vi "Axsun GUI.vi"() -> ()   [LabVIEW 2018]
uses:
  cluster_Axsun.ctl
  General/Controls/Queue Manager Actions.ctl
  General/Controls/MessagePacket.ctl
  Axsun action.ctl
panel:
  in  "stop":bool
  out "error out":errorcluster
  out "output cluster":T1={"device array"=[], "control version"="", "Serial num"="A18009851", "LaserONTime"=0, "wave length\nat trigger"=0.0, "System status"=0.0, "clock delay"=0}
  in  "Source OFF":bool
  in  "Source ON":bool
  in  "Laser OFF":bool
  in  "Laser ON":bool
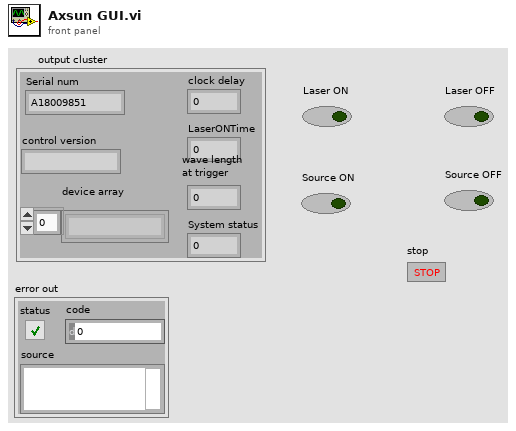
[diagram p1: front panel]
types:
  T1 = typedef "cluster_Axsun.ctl" = cluster{"device array":string[], "control version":string, "Serial num":string, "LaserONTime":i32, "wave length\nat trigger":dbl, "System status":dbl, "clock delay":u32}
  T2 = typedef "MessagePacket.ctl" = cluster{"Message":string, "Parameter":variant}
  T3 = typedef "Queue Manager Actions.ctl" = enum16{"Init", "Enqueue", "Enqueue All", "Preview Queue", "Dequeue", "Get Status", "Flush Queue", "Flush All Queues", "Release All Queues", "Release Queue", "Enqueue at Opposite End"}
  T4 = typedef "Axsun action.ctl" = enum16{"GetSystemStatus", "Clock delay", "GetLaserOnTime", "GetWaveLengthAtSweptTrigger", "Source current ON", "GetSerialNum", "GetControlVersion", "Laser ON", "Laser OFF", "Source current OFF", "Get laser handle", "Start Network Control Interface", "stop", "Create handle"}
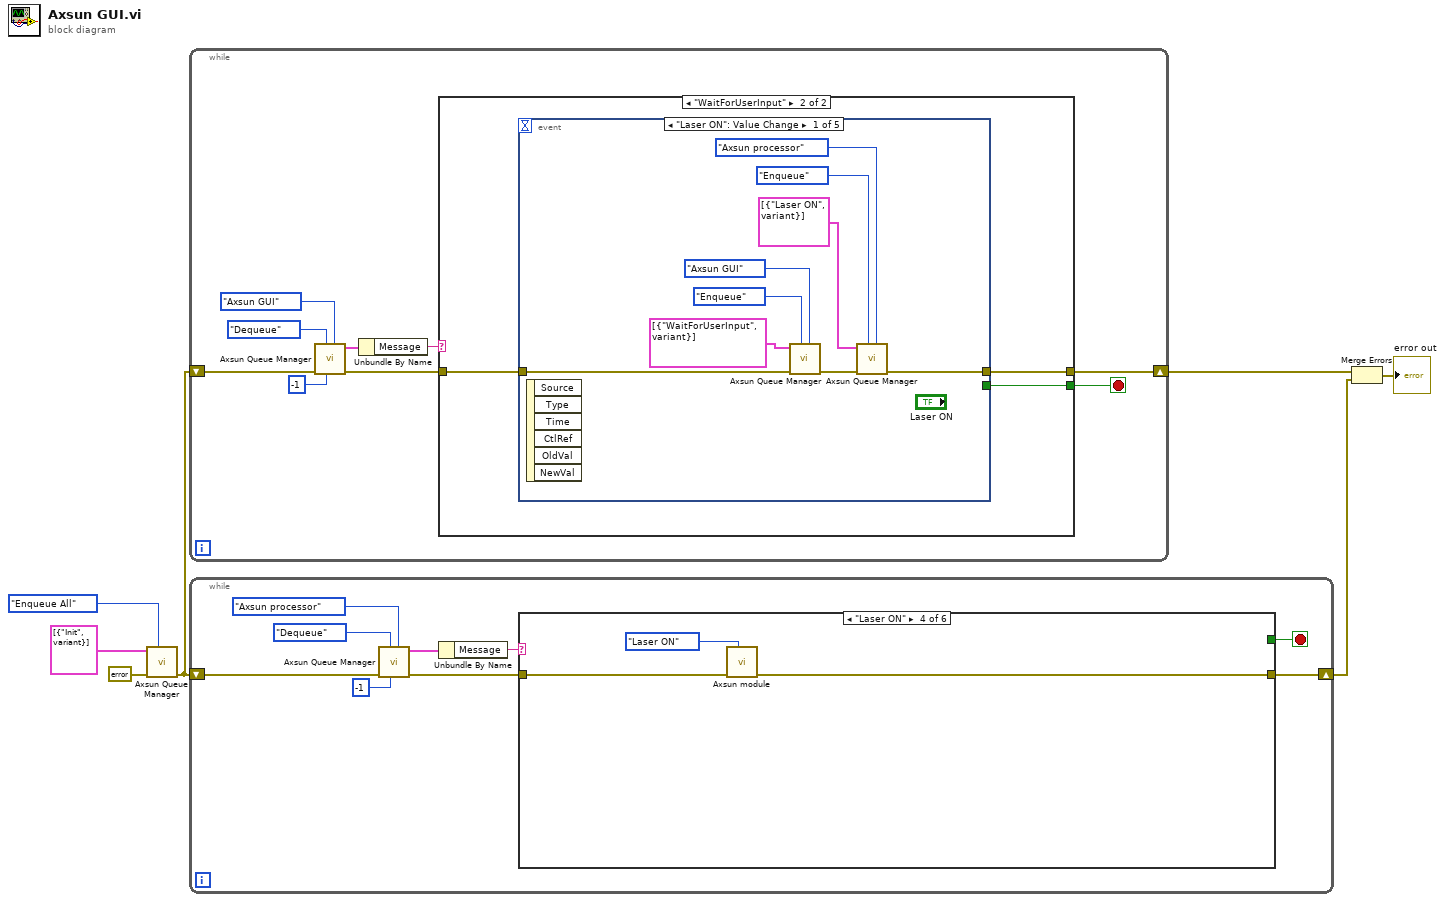
[diagram p0: block diagram]
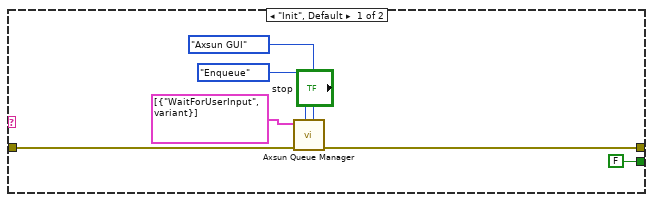
[diagram p2: hidden frame]
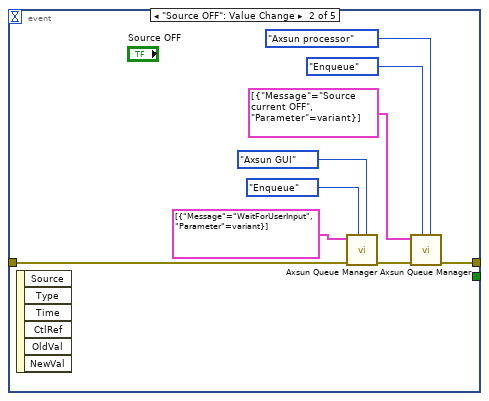
[diagram p3: hidden frame]
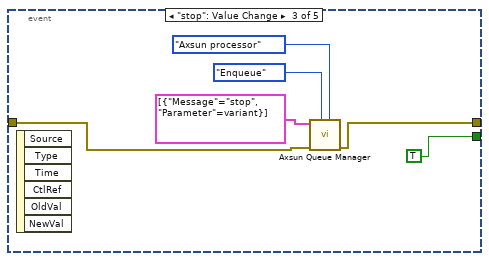
[diagram p4: hidden frame]
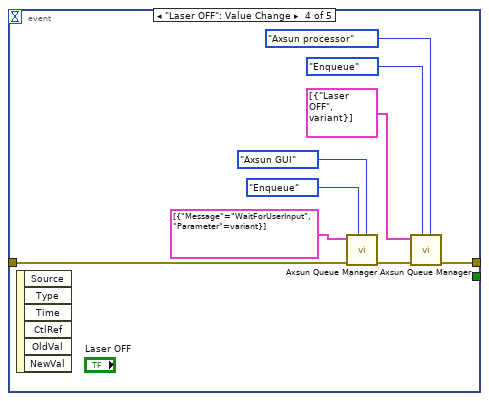
[diagram p5: hidden frame]
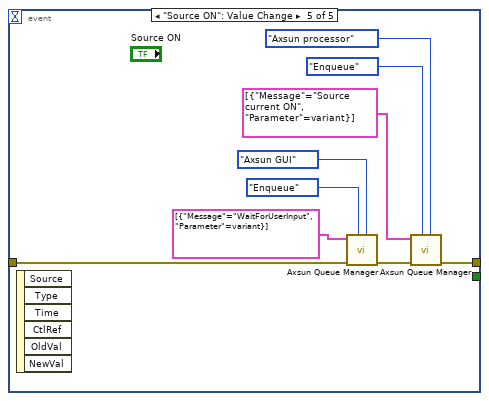
[diagram p6: hidden frame]
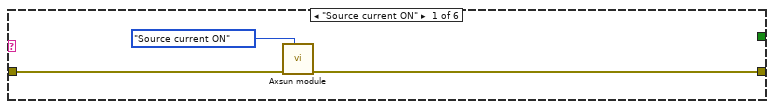
[diagram p7: hidden frame]
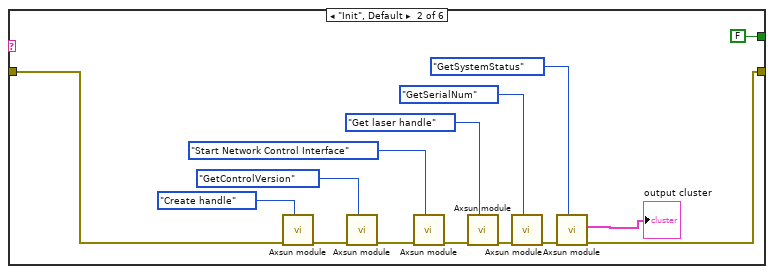
[diagram p8: hidden frame]
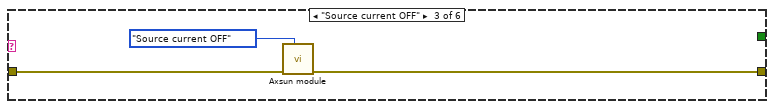
[diagram p9: hidden frame]
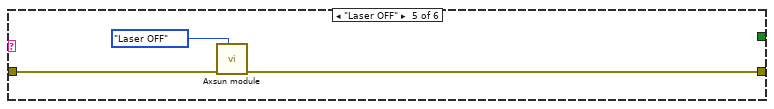
[diagram p10: hidden frame]
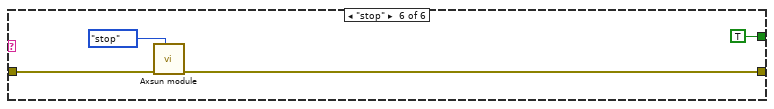
[diagram p11: hidden frame]
diagram:
  n1 = call "Axsun Queue Manager.vi"("Action"=Queue_Manager_Actions."Enqueue All", "Error In"=errorcluster {"status"=FALSE, "code"=0, "source"=""} ("error in (no error)"), "Message Packet Array"=T2[] [{"Message"="Init", "Parameter"=variant}]) -> ("Error Out"=w4:errorcluster)  [unwired: 5 in, 3 out]
  n2 = while {
    shift-right: [w11] -> w3
    shift-left: w4 -> [w13]
    stop <- w10 stop-if-true
    n3 = call "Axsun Queue Manager.vi"("queue name"=enum16{"Axsun processor", "Axsun GUI"}."Axsun GUI", "timeout in ms (-1)"=-1, "Action"=Queue_Manager_Actions."Dequeue", "Error In"=w13) -> ("Error Out"=w12:errorcluster, "Message Packet [Out]"=w14:T2)  [unwired: 4 in, 2 out]
    n4 = Unbundle By Name(w14) -> ("Message"=w9:string)
    n5 = case shown="\"WaitForUserInput\"" w9 {
      tunnel: w12 -> [w22 w25]
      tunnel: [w21 w24] -> w11
      tunnel: [FALSE w23] -> w10
      frame "Init", Default {
        n6 = call "Axsun Queue Manager.vi"("queue name"=enum16{"Axsun processor", "Axsun GUI"}."Axsun GUI", "Action"=Queue_Manager_Actions."Enqueue", "Error In"=w22, "Message Packet Array"=T2[] [{"Message"="WaitForUserInput", "Parameter"=variant}]) -> ("Error Out"=w21:errorcluster)  [unwired: 4 in, 3 out]
      }
      frame "WaitForUserInput" {
        n7 = event shown="[0] \"Laser ON\": Value Change" {
          selector: _ -> [_ _ _ _ _]
          dyn-events: _ -> [_ _ _ _ _]
          timeout: _ -> [_ _ _ _ _]
          tunnel: w25 -> [w34 w36 w46 w52 w61]
          tunnel: [w32 w35 w45 w50 w59] -> w24
          tunnel: [_ _ TRUE _ _] -> w23
          event "Laser ON": Value Change {
            n8 = event-data() -> ()  [unwired: 1 in, 6 out]
            n9 = call "Axsun Queue Manager.vi"("queue name"=enum16{"Axsun processor", "Axsun GUI"}."Axsun GUI", "Action"=Queue_Manager_Actions."Enqueue", "Error In"=w34, "Message Packet Array"=T2[] [{"Message"="WaitForUserInput", "Parameter"=variant}]) -> ("Error Out"=w33:errorcluster)  [unwired: 4 in, 3 out]
            n10 = call "Axsun Queue Manager.vi"("queue name"=enum16{"Axsun processor", "Axsun GUI"}."Axsun processor", "Action"=Queue_Manager_Actions."Enqueue", "Error In"=w33, "Message Packet Array"=T2[] [{"Message"="Laser ON", "Parameter"=variant}]) -> ("Error Out"=w32:errorcluster)  [unwired: 4 in, 3 out]
          }
          event "Source OFF": Value Change {
            n11 = event-data() -> ()  [unwired: 1 in, 6 out]
            n12 = call "Axsun Queue Manager.vi"("queue name"=enum16{"Axsun processor", "Axsun GUI"}."Axsun GUI", "Action"=Queue_Manager_Actions."Enqueue", "Error In"=w36, "Message Packet Array"=T2[] [{"Message"="WaitForUserInput", "Parameter"=variant}] ("Message Packet [In]")) -> ("Error Out"=w43:errorcluster)  [unwired: 4 in, 3 out]
            n13 = call "Axsun Queue Manager.vi"("queue name"=enum16{"Axsun processor", "Axsun GUI"}."Axsun processor", "Action"=Queue_Manager_Actions."Enqueue", "Error In"=w43, "Message Packet Array"=T2[] [{"Message"="Source current OFF", "Parameter"=variant}]) -> ("Error Out"=w35:errorcluster)  [unwired: 4 in, 3 out]
          }
          event "stop": Value Change {
            n14 = event-data() -> ()  [unwired: 1 in, 6 out]
            n15 = call "Axsun Queue Manager.vi"("queue name"=enum16{"Axsun processor", "Axsun GUI"}."Axsun processor", "Action"=Queue_Manager_Actions."Enqueue", "Error In"=w46, "Message Packet Array"=T2[] [{"Message"="stop", "Parameter"=variant}]) -> ("Error Out"=w45:errorcluster)  [unwired: 4 in, 3 out]
          }
          event "Laser OFF": Value Change {
            n16 = event-data() -> ()  [unwired: 1 in, 6 out]
            n17 = call "Axsun Queue Manager.vi"("queue name"=enum16{"Axsun processor", "Axsun GUI"}."Axsun GUI", "Action"=Queue_Manager_Actions."Enqueue", "Error In"=w52, "Message Packet Array"=T2[] [{"Message"="WaitForUserInput", "Parameter"=variant}] ("Message Packet [In]")) -> ("Error Out"=w58:errorcluster)  [unwired: 4 in, 3 out]
            n18 = call "Axsun Queue Manager.vi"("queue name"=enum16{"Axsun processor", "Axsun GUI"}."Axsun processor", "Action"=Queue_Manager_Actions."Enqueue", "Error In"=w58, "Message Packet Array"=T2[] [{"Message"="Laser OFF", "Parameter"=variant}]) -> ("Error Out"=w50:errorcluster)  [unwired: 4 in, 3 out]
          }
          event "Source ON": Value Change {
            n19 = event-data() -> ()  [unwired: 1 in, 6 out]
            n20 = call "Axsun Queue Manager.vi"("queue name"=enum16{"Axsun processor", "Axsun GUI"}."Axsun GUI", "Action"=Queue_Manager_Actions."Enqueue", "Error In"=w61, "Message Packet Array"=T2[] [{"Message"="WaitForUserInput", "Parameter"=variant}] ("Message Packet [In]")) -> ("Error Out"=w67:errorcluster)  [unwired: 4 in, 3 out]
            n21 = call "Axsun Queue Manager.vi"("queue name"=enum16{"Axsun processor", "Axsun GUI"}."Axsun processor", "Action"=Queue_Manager_Actions."Enqueue", "Error In"=w67, "Message Packet Array"=T2[] [{"Message"="Source current ON", "Parameter"=variant}]) -> ("Error Out"=w59:errorcluster)  [unwired: 4 in, 3 out]
          }
        }
      }
    }
  }
  n22 = while {
    shift-right: [w70] -> w2
    shift-left: w4 -> [w76]
    stop <- w69 stop-if-true
    n23 = call "Axsun Queue Manager.vi"("queue name"=enum16{"Axsun processor", "Axsun GUI"}."Axsun processor", "timeout in ms (-1)"=-1, "Action"=Queue_Manager_Actions."Dequeue", "Error In"=w76) -> ("Error Out"=w75:errorcluster, "Message Packet [Out]"=w72:T2)  [unwired: 4 in, 2 out]
    n24 = Unbundle By Name(w72) -> ("Message"=w71:string)
    n25 = case shown="\"Laser ON\"" w71 {
      tunnel: w75 -> [w79 w83 w96 w99 w102 w106]
      tunnel: [w78 w81 w95 w98 w101 w105] -> w70
      tunnel: [_ FALSE _ _ _ TRUE] -> w69
      frame "Source current ON" {
        n26 = call "Axsun module.vi"("Action"=Axsun_action."Source current ON", "error in (no error)"=w79) -> ("error out"=w78:errorcluster)  [unwired: 8 in, 1 out]
      }
      frame "Init", Default {
        n27 = call "Axsun module.vi"("Action"=Axsun_action."Create handle", "error in (no error)"=w83) -> ("error out"=w93:errorcluster)  [unwired: 8 in, 1 out]
        n28 = call "Axsun module.vi"("Action"=Axsun_action."GetControlVersion", "error in (no error)"=w93) -> ("error out"=w92:errorcluster)  [unwired: 8 in, 1 out]
        n29 = call "Axsun module.vi"("Action"=Axsun_action."Start Network Control Interface", "error in (no error)"=w92) -> ("error out"=w91:errorcluster)  [unwired: 8 in, 1 out]
        n30 = call "Axsun module.vi"("Action"=Axsun_action."Get laser handle", "error in (no error)"=w91) -> ("error out"=w90:errorcluster)  [unwired: 8 in, 1 out]
        n31 = call "Axsun module.vi"("Action"=Axsun_action."GetSerialNum", "error in (no error)"=w90) -> ("error out"=w89:errorcluster)  [unwired: 8 in, 1 out]
        n32 = call "Axsun module.vi"("Action"=Axsun_action."GetSystemStatus", "error in (no error)"=w89) -> ("error out"=w81:errorcluster, "output cluster"=→"output cluster":T1)  [unwired: 8 in]
      }
      frame "Source current OFF" {
        n33 = call "Axsun module.vi"("Action"=Axsun_action."Source current OFF", "error in (no error)"=w96) -> ("error out"=w95:errorcluster)  [unwired: 8 in, 1 out]
      }
      frame "Laser ON" {
        n34 = call "Axsun module.vi"("Action"=Axsun_action."Laser ON", "error in (no error)"=w99) -> ("error out"=w98:errorcluster)  [unwired: 8 in, 1 out]
      }
      frame "Laser OFF" {
        n35 = call "Axsun module.vi"("Action"=Axsun_action."Laser OFF", "error in (no error)"=w102) -> ("error out"=w101:errorcluster)  [unwired: 8 in, 1 out]
      }
      frame "stop" {
        n36 = call "Axsun module.vi"("Action"=Axsun_action."stop", "error in (no error)"=w106) -> ("error out"=w105:errorcluster)  [unwired: 8 in, 1 out]
      }
    }
  }
  n37 = Merge Errors(w3, w2) -> (→"error out":errorcluster)
